vi "Init PublicEvents.vi"(8 "error in (no error)":errorcluster, 10 "SMO":refnum<class "SMO.lvclass">, 11 "PublicEvents":refnum<class "PublicEvents.lvclass">) -> (0 "error out":errorcluster, 3 "PublicEvents":refnum<class "PublicEvents.lvclass">)   [LabVIEW 2013, in "SMOFacade.lvlib" / "PublicEvents.lvclass"]
uses:
  PublicEvents.lvclass
  SMO/SMO.lvclass
  PublicEvents.lvclass/PublicEvents.ctl
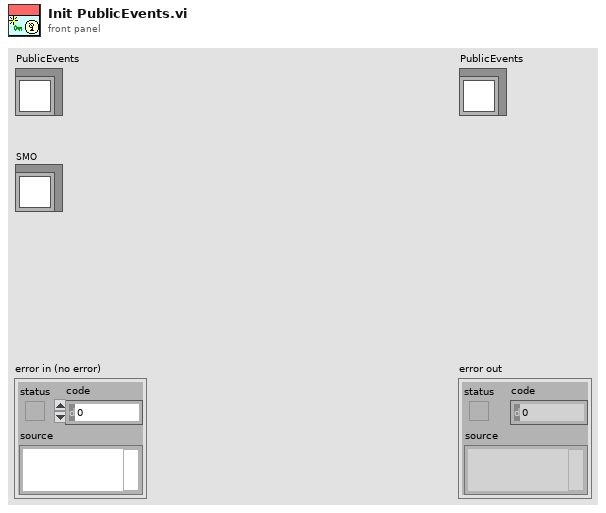
[diagram p1: front panel]
types:
  T1 = typedef "SMO.lvclass/Public Events.ctl" = cluster{"Error":refnum<user-event>, "State":refnum<user-event>, "Reserve State":refnum<user-event>}
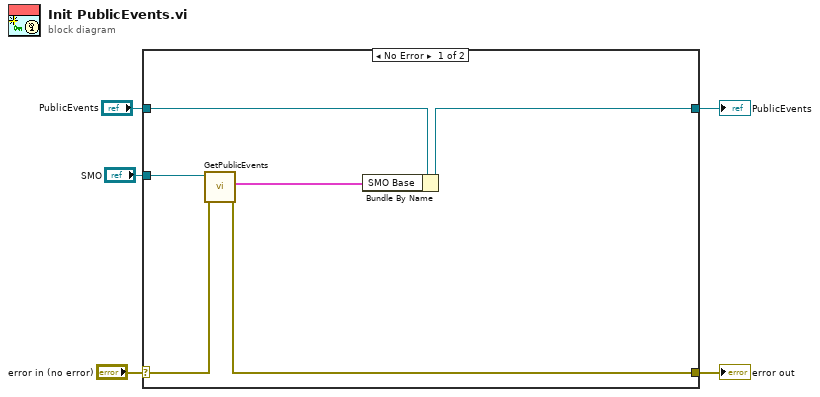
[diagram p0: block diagram]
diagram:
  n1 = case shown="No Error" "error in (no error)" {
    selector: "error in (no error)" -> [w7 w13]
    tunnel: [w6 w13] -> w4
    tunnel: [w10 w12] -> w3
    tunnel: "PublicEvents" -> [w11 w12]
    tunnel: "SMO" -> [w9 _]
    frame No Error {
      n2 = call "GetPublicEvents.vi"("error in (no error)"=w7, "SMO"=w9) -> ("error out"=w6:errorcluster, "Public Events"=w8:T1)  [unwired: 7 in, 1 out]
      n3 = Bundle By Name(cluster=w11, "SMO Base"=w8) -> (w10:refnum<class "PublicEvents.lvclass">)
    }
    frame Error {
    }
  }
  "error out" <- w4
  "PublicEvents" <- w3
